vi "Global_InitEndSync.vi"() -> ()   [LabVIEW 2017]
panel:
  out "Reset Movie":bool
  in  "Top Button":bool
  in  "Play":bool
  out "Finish":bool
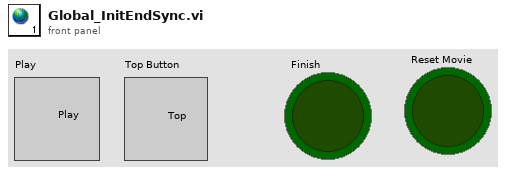
[diagram p1: front panel]
diagram:
